vi "Unit Test Preserve wired non-serialized data (Expansion) False.vi"() -> ()   [LabVIEW 2019, in "Sports Unit Tests.lvclass"]
uses:
  Sports Unit Tests.lvclass
  <vilib>/addons/_JKI Toolkits/Caraya/classes/Assert/Assert.lvclass
  Classes/Adam Sandler/Adam Sandler.lvclass
  <vilib>/addons/_JKI Toolkits/Caraya/classes/Assert/Assert Equal Value_Variant.vi
  <vilib>/addons/_JKI Toolkits/Caraya/classes/Assert/Assert Not Error.vi
  Classes/Sports Player/Sports Player.lvclass
  <userlib>/Blue Origin/BlueSerialization/BlueSerializer/DeserializeMutationOptions.ctl
  <userlib>/Blue Origin/BlueSerialization/BlueSerializer/BlueSerializer.lvclass
  <userlib>/Blue Origin/BlueSerialization/BlueSerializer/DeserializeSlicingOptions.ctl
  <userlib>/Blue Origin/BlueSerialization/BlueSerializer/DeserializeOptions.ctl
  <userlib>/Blue Origin/BlueSerialization/BlueSerializer/DeserializePreservationOptions.ctl
  <userlib>/Blue Origin/BlueSerialization/BlueSerializer/PreserveNonWiredDataOption.ctl
panel:
  out "Table":string[][](table)
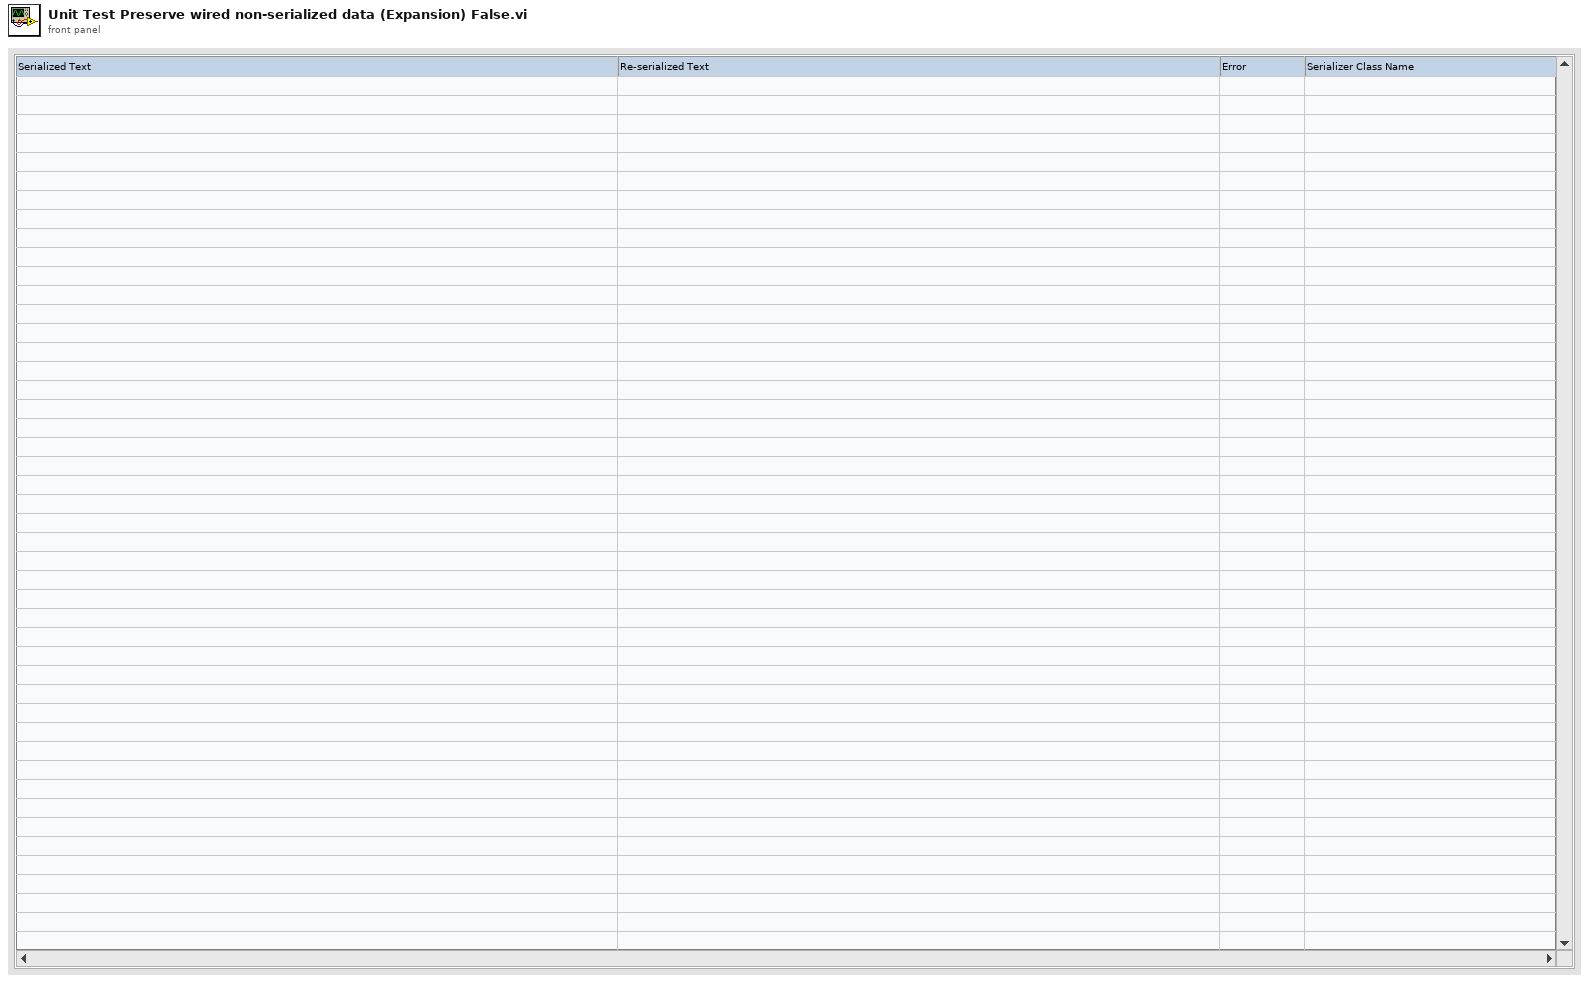
[diagram p1: front panel]
types:
  T1 = typedef "BlueSerialization.lvlib/BlueSerializer.lvclass/PreserveNonWiredDataOption.ctl" = enum16{"Don't preserve", "Preserve (error on less-specific wired types)", "Preserve (except on less-specific wired types)"}
  T2 = typedef "BlueSerialization.lvlib/BlueSerializer.lvclass/DeserializeOptions.ctl" = cluster{"deserialize non-BlueSerializable objects from hex?":bool, "expand objects on type conflict?":bool, "Slicing":T3, "Mutation Options":T4, "Preservation Options":T5}
  T3 = typedef "BlueSerialization.lvlib/BlueSerializer.lvclass/DeserializeSlicingOptions.ctl" = cluster{"slice flattened object data on error?":bool, "sliceable class names":string[]}
  T4 = typedef "BlueSerialization.lvlib/BlueSerializer.lvclass/DeserializeMutationOptions.ctl" = cluster{"error on inserted parent levels?":bool, "\terror on obsolete parent levels?":bool}
  T5 = typedef "BlueSerialization.lvlib/BlueSerializer.lvclass/DeserializePreservationOptions.ctl" = cluster{"Preserve wired serialized data?":bool, "Preserve wired non-serialized data":T1}
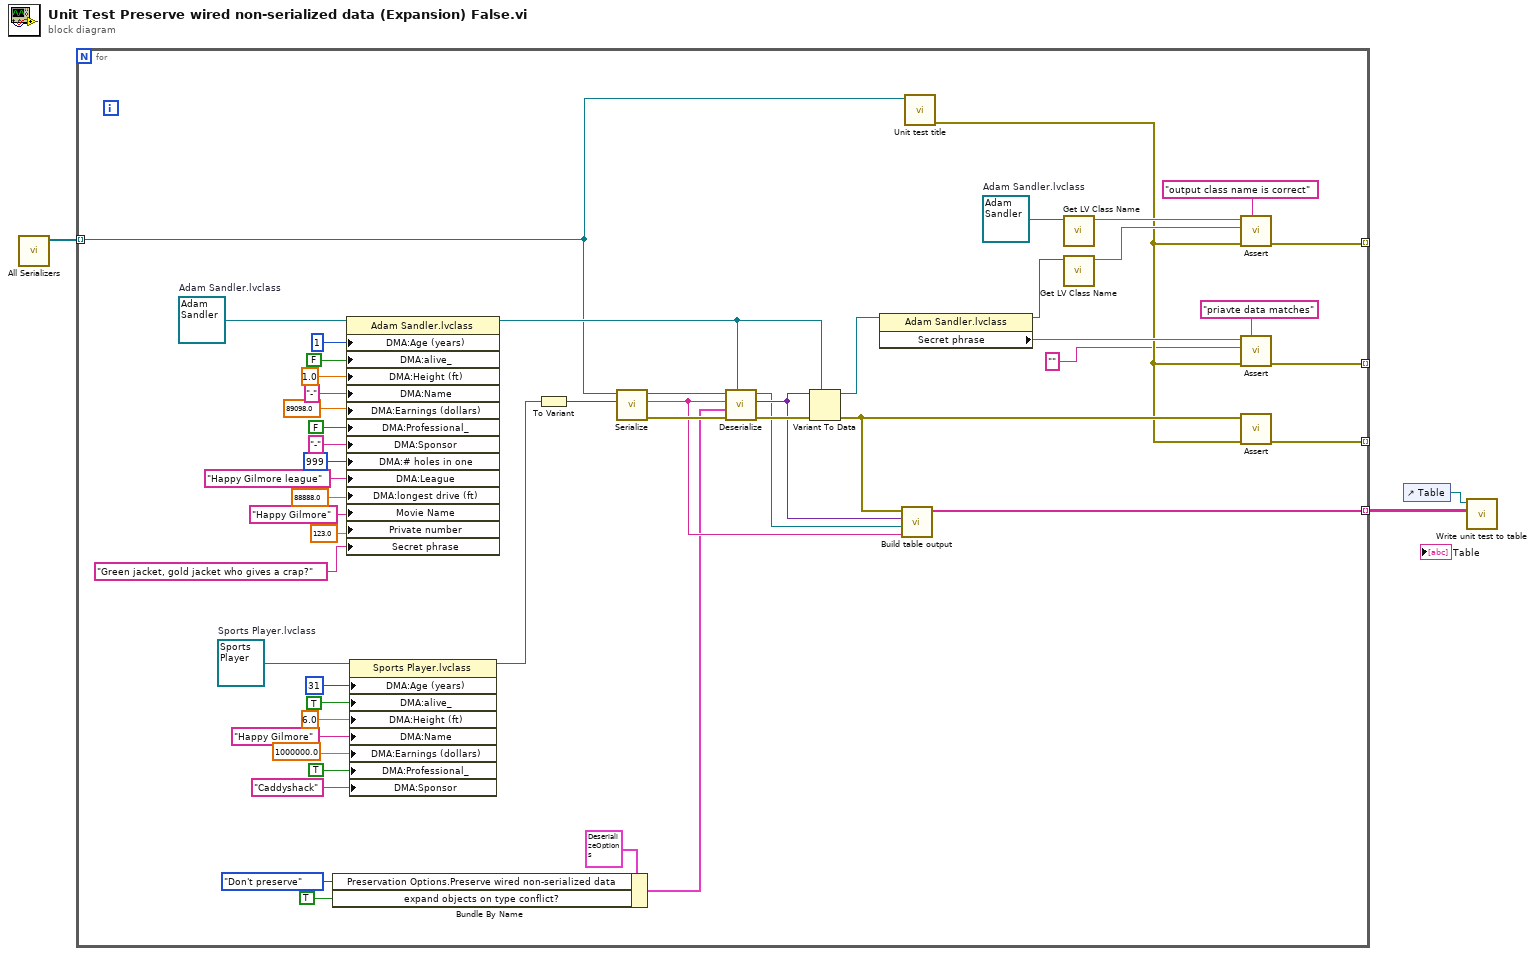
[diagram p0: block diagram]
diagram:
  n1 = call "All Serializers.vi"() -> ("All serializers"=w2:refnum<class "BlueSerializer.lvclass">[])  [unwired: 11 in]
  n2 = for {
    tunnel: w2 -> [w5] mode=indexing
    tunnel: [w40] -> _ mode=indexing
    tunnel: [w39] -> _ mode=indexing
    tunnel: [w34] -> w1 mode=indexing
    tunnel: [w20] -> _ mode=indexing
    w17 = refnum<class "Sports Player.lvclass"> refnum  # Sports Player.lvclass
    w27 = refnum<class "Adam Sandler.lvclass"> refnum  # Adam Sandler.lvclass
    w33 = refnum<class "Adam Sandler.lvclass"> refnum  # Adam Sandler.lvclass
    n3 = Bundle By Name(cluster=T2 {"deserialize non-BlueSerializable objects from hex?"=FALSE, "expand objects on type conflict?"=FALSE, "Slicing"={"slice flattened object data on error?"=FALSE, "sliceable class names"=[]}, "Mutation Options"={"error on inserted parent levels?"=FALSE, "\terror on obsolete parent levels?"=FALSE}, "Preservation Options"={"Preserve wired serialized data?"=FALSE, "Preserve wired non-serialized data"=enum."Don't preserve"}} ("Deserialize Options"), "Preservation Options.Preserve wired non-serialized data"=PreserveNonWiredDataOption."Don't preserve", "expand objects on type conflict?"=TRUE ("Allow class expansion?")) -> (w6:T2)
    n4 = property on="Property Node" class="Adam Sandler.lvclass"(reference=w33, "DMA:Age (years)"=u16 1 ("Age (years)"), "DMA:alive_"=FALSE ("alive_"), "DMA:Height (ft)"=1.0 ("Height (ft)"), "DMA:Name"="-" ("Name"), "DMA:Earnings (dollars)"=89098.0 ("Earnings (dollars)"), "DMA:Professional_"=FALSE ("Professional_"), "DMA:Sponsor"="-" ("Sponsor"), "DMA:# holes in one"=999 ("# holes in one"), "DMA:League"="Happy Gilmore league" ("League"), "DMA:longest drive (ft)"=88888.0 ("longest drive (ft)"), "Movie Name"="Happy Gilmore", "Private number"=123.0, "Secret phrase"="Green jacket, gold jacket who gives a crap?") -> (reference out=w19:refnum<class "Adam Sandler.lvclass">)  [unwired: 1 in, 1 out]
    n5 = property on="Property Node" class="Sports Player.lvclass"(reference=w17, "DMA:Age (years)"=u16 31 ("Age (years)"), "DMA:alive_"=TRUE ("alive_"), "DMA:Height (ft)"=6.0 ("Height (ft)"), "DMA:Name"="Happy Gilmore" ("Name"), "DMA:Earnings (dollars)"=1000000.0 ("Earnings (dollars)"), "DMA:Professional_"=TRUE ("Professional_"), "DMA:Sponsor"="Caddyshack" ("Sponsor")) -> (reference out=w9:refnum<class "Sports Player.lvclass">)  [unwired: 1 in, 1 out]
    n6 = To Variant(anything=w9) -> (Variant=w52:variant)
    n7 = call <userlib>:"Serialize.vi"("Anything"=w52, "BlueSerializer in"=w5) -> ("error out"=w54:errorcluster, "Serialized Text"=w35:string, "BlueSerializer out"=w53:refnum<class "BlueSerializer.lvclass">)  [unwired: 7 in]
    n8 = call <userlib>:"Deserialize.vi"("Anything"=w19, "error in (no error)"=w54, "Deserialize Options"=w6, "Serialized Text"=w35, "BlueSerializer in"=w53) -> ("error out"=w51:errorcluster, "Variant"=w37:variant, "BlueSerializer out"=w36:refnum<class "BlueSerializer.lvclass">)  [unwired: 4 in]
    n9 = Variant To Data(error in=w51, type=w19, Variant=w37) -> (data=w25:refnum<class "Adam Sandler.lvclass">, error out=w38:errorcluster)
    n10 = property class="Adam Sandler.lvclass"(reference=w25) -> (reference out=w24:refnum<class "Adam Sandler.lvclass">, "Secret phrase"=w23:string)  [unwired: 1 in, 1 out]
    n11 = call "Build table output.vi"("serialized text"=w35, "BlueSerializer in"=w36, "deserialized variant"=w37, "variant to data error"=w38) -> ("table output"=w34:string[])  [unwired: 7 in]
    n12 = call "Unit test title.vi"("serializer"=w5) -> ("error out"=w21:errorcluster)  [unwired: 9 in, 1 out]
    n13 = call <vilib>:"Get LV Class Name.vi"("object"=w27) -> ("class name"=w50:string)  [unwired: 9 in, 1 out]
    n14 = call <vilib>:"Get LV Class Name.vi"("object"=w24) -> ("class name"=w49:string)  [unwired: 9 in, 1 out]
    n15 = call-poly <vilib>:"Assert.vi"("Label"="output class name is correct", "error in (no error)"=w21, "Y"=w49, "X"=w50) -> ("error out"=w39:errorcluster)  [unwired: 7 in]
    n16 = call-poly <vilib>:"Assert.vi"("Label"="priavte data matches", "error in (no error)"=w21, "Y"="" ("Secret phrase"), "X"=w23) -> ("error out"=w20:errorcluster)  [unwired: 7 in]
    n17 = call-poly <vilib>:"Assert.vi"("error in (no error)"=w21, "Not Error?"=w38) -> ("error out"=w40:errorcluster)  [unwired: 9 in]
  }
  n18 = control-ref of="Table"() -> (w3:refnum<vi>)
  n19 = call "Write unit test to table.vi"("Table"=w1, "Table ref in"=w3) -> ()  [unwired: 9 in, 1 out]
